vi "UnscentedKalmanFilter_SetP.vi"(10 "P":T1, 11 "in UnscentedKalmanFiilter":T2) -> (0 "SizeCoerced":bool, 3 "out UnscentedKalmanFiilter":T2)   [LabVIEW 2019, in "Trajectory_Library.lvlib"]
doc: "Sets the entire error covariance matrix P.\n \nInputs:\n - inUnscentedKalmanFilter -- filter data cluster\n - newP -- The new value of P to use.\n\nOutputs:\n - outUnscentedKalmanFilter -- updated filter data cluster\n - sizeCoerced -- If TRUE, an error occured"
uses:
  Trajectory_Library.lvlib
  UNSCENTED_KALMAN_FILTER.ctl
  <vilib>/Analysis/Matrix/Datatypes/RealMatrix.ctl
  MERWE_SCALED_SIGMA_PTS.ctl
  BiFun_Matrix_FUNC_TYPE.ctl
  MatBuilder_Create.vi
  <vilib>/Analysis/Matrix/NI_Matrix.lvlib
panel:
  # "State Estimate <Statess,1>"
  # "<States, States>"
  # "<States, ?>"
  # "<Statess,  States>"
  # "<Outputs, Outputs>"
  # "<?, 1>"
  # "<?, 1>"
  # "State Estimate <Statess,1>"
  # "<States, States>"
  # "<States, ?>"
  # "<Statess,  States>"
  # "<Outputs, Outputs>"
  # "<?, 1>"
  # "<?, 1>"
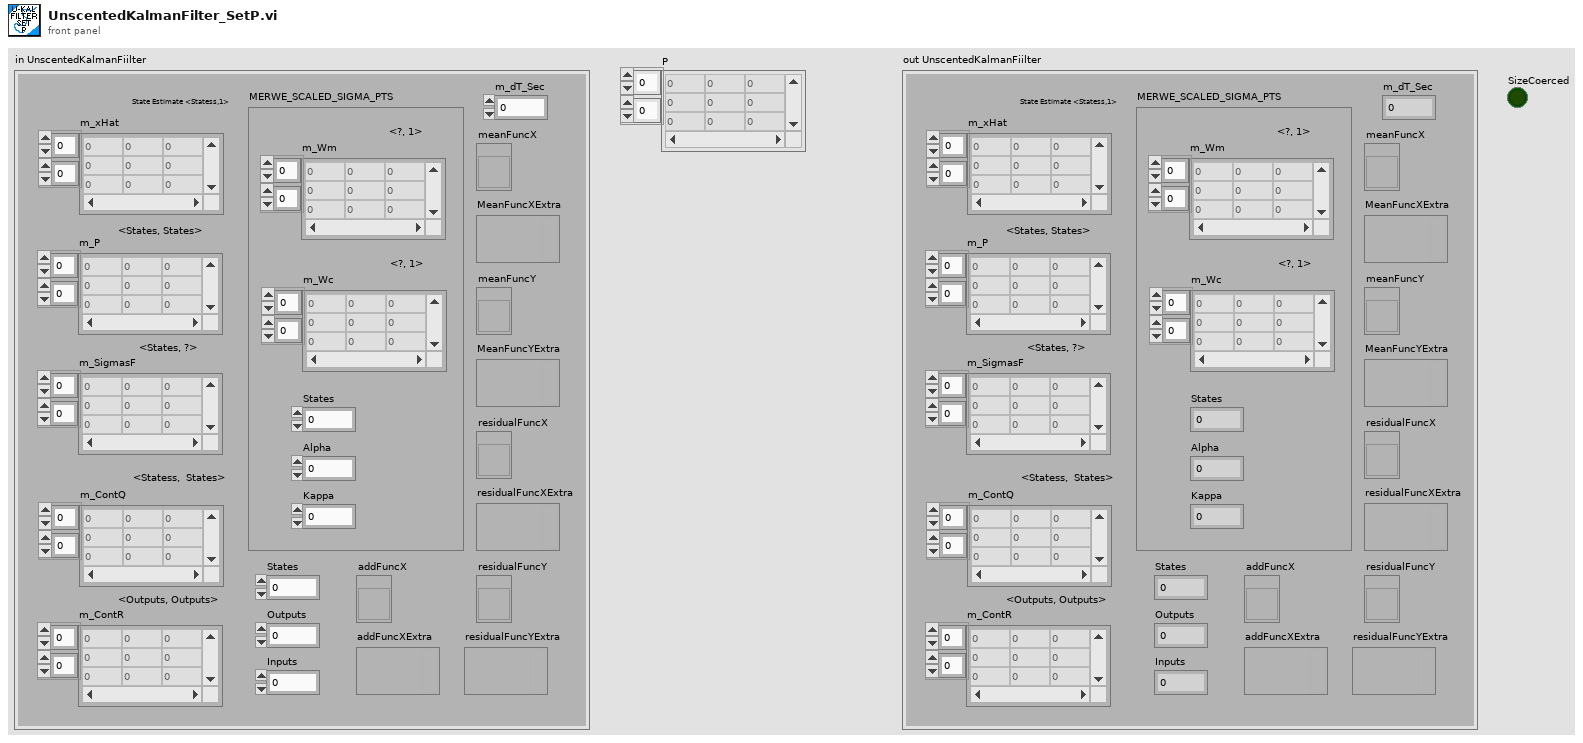
[diagram p1: front panel]
types:
  T1 = typedef "NI_Matrix.lvlib/RealMatrix.ctl" = dbl[][]
  T2 = typedef "Trajectory_Library.lvlib/UNSCENTED_KALMAN_FILTER.ctl" = cluster{"m_P":T1, "m_xHat":T1, "States":i32, "Outputs":i32, "m_ContR":T1, "m_ContQ":T1, "m_SigmasF":T1, "m_dT_Sec":dbl, "MERWE_SCALED_SIGMA_PTS":T3, "meanFuncX":T4, "meanFuncY":T4, "residualFuncX":T4, "residualFuncY":T4, "addFuncX":T4, "addFuncXExtra":variant, "residualFuncYExtra":variant, "residualFuncXExtra":variant, "MeanFuncYExtra":variant, "MeanFuncXExtra":variant, "Inputs":i32}
  T3 = typedef "Trajectory_Library.lvlib/MERWE_SCALED_SIGMA_PTS.ctl" = cluster{"m_Wm":T1, "States":i32, "Alpha":dbl, "m_Wc":T1, "Kappa":i32}
  T4 = typedef "Trajectory_Library.lvlib/BiFun_Matrix_FUNC_TYPE.ctl" = refnum<vi>
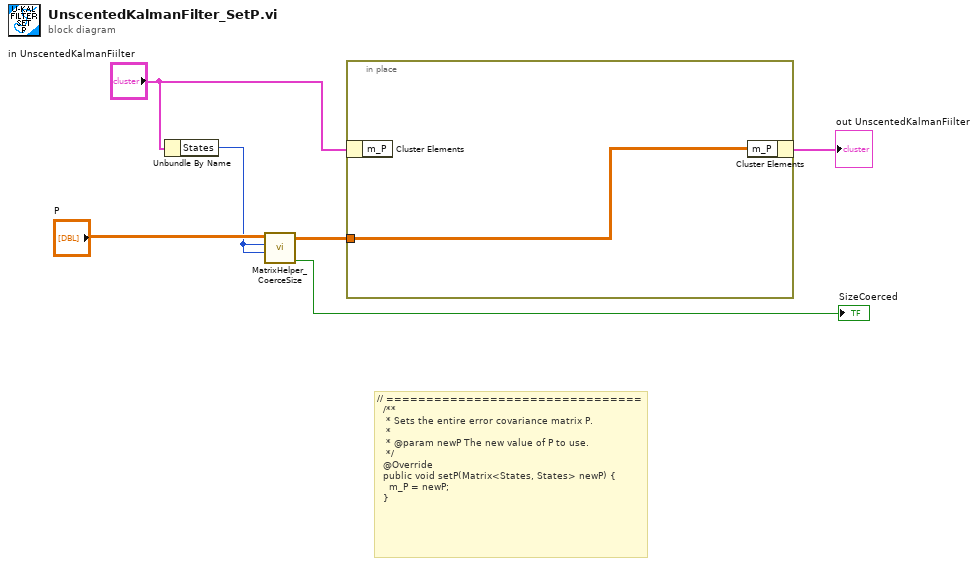
[diagram p0: block diagram]
diagram:
  # "// ================================\n  /**\n   * Sets the entire error covariance matrix P.\n   *\n   * @param newP The new value of P to use.\n   */\n  @Override\n  public void setP(Matrix<States, States> newP) {\n    m_P = newP;\n  }"
  n1 = Unbundle By Name("in UnscentedKalmanFiilter") -> ("States"=w3:i32)
  n2 = call "MatrixHelper_CoerceSize.vi"("Columns"=w3, "Rows"=w3, "input matrix"="P") -> ("Coerced"=→"SizeCoerced":bool, "output matrix"=w5:T1)  [unwired: 7 in]
  n3 = in-place {
    in-place-border: w5 -> [w7]
    n4 = in-place-cluster #1("in UnscentedKalmanFiilter") -> ()  [unwired: 1 out]
    n5 = in-place-cluster #1("m_P"=w7) -> (→"out UnscentedKalmanFiilter":T2)
  }
